vi "Set Variables.vi"(8 "error in (no error)":errorcluster, 10 "Variables":variant, 11 "Bitwise Popup in":refnum<class "Bitwise Functions.lvclass">) -> (0 "error out":errorcluster, 3 "Bitwise Popup out":refnum<class "Bitwise Functions.lvclass">)   [LabVIEW 2016, in "Bitwise Functions.lvclass"]
uses:
  Bitwise Functions.lvclass
  Bitwise Functions.lvclass/Bitwise Functions.ctl
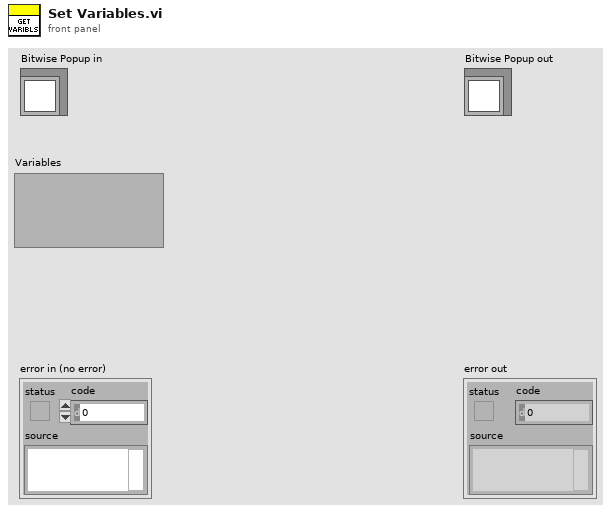
[diagram p1: front panel]
types:
  T1 = typedef "Bitwise Functions.lvclass/Variables.ctl" = cluster{"Var1":variant, "Var2":variant}
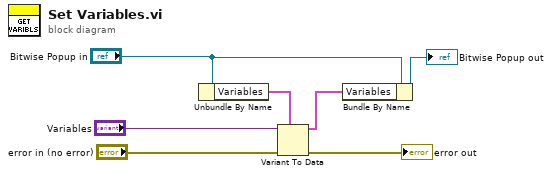
[diagram p0: block diagram]
diagram:
  n1 = Unbundle By Name("Bitwise Popup in") -> ("Variables"=w2:T1)
  n2 = Variant To Data(error in="error in (no error)", type=w2, Variant="Variables") -> (data=w1:T1, error out=→"error out":errorcluster)
  n3 = Bundle By Name(cluster="Bitwise Popup in", "Variables"=w1) -> (→"Bitwise Popup out":refnum<class "Bitwise Functions.lvclass">)
